vi "tcpwritendata.vi"(8 "error in (no error)":errorcluster, 9 "timeout ms (25000)":i32=25000, 10 "data in":string, 11 "refnum in":refnum<k5>) -> (0 "error out":errorcluster, 2 "bytes written":i32, 3 "refnum out":refnum<k5>)   [LabVIEW 2012]
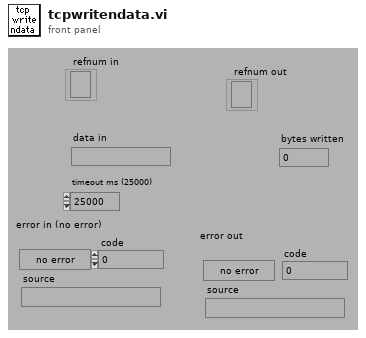
[diagram p1: front panel]
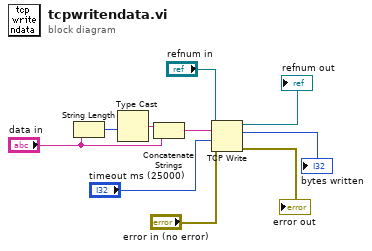
[diagram p0: block diagram]
diagram:
  n1 = String Length(string="data in") -> (length=w9:i32)
  n2 = Type Cast(x=w9) -> (*(type *) &x=w7:string)  [unwired: 1 in]
  n3 = Concatenate Strings(w7, "data in") -> (w10:string)
  n4 = TCP Write(connection ID="refnum in", data in=w10, error in (no error)="error in (no error)", 9:"timeout ms (25000)") -> (connection ID out=→"refnum out":refnum<k5>, bytes written=→"bytes written":i32, error out=→"error out":errorcluster)
